vi "NT4 Format Generic  to String.vi"(9 "Quote Elements":bool, 11 "Variant":variant) -> (2 "Type String":string, 3 "String":string)   [LabVIEW 2025]
doc: "Format the generic union data into a string."
uses:
  <vilib>/Rock Robotics/Network Tables/NT Datatype.ctl
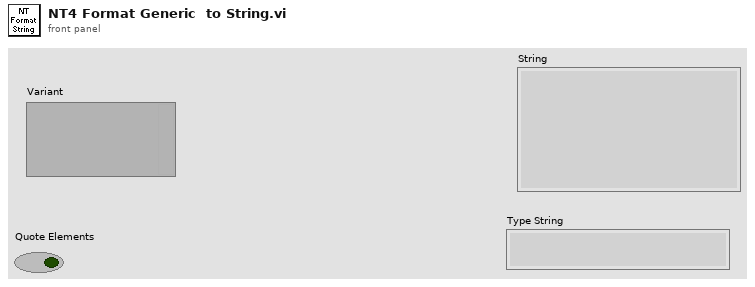
[diagram p1: front panel]
types:
  T1 = typedef "NT Datatype.ctl" = u32
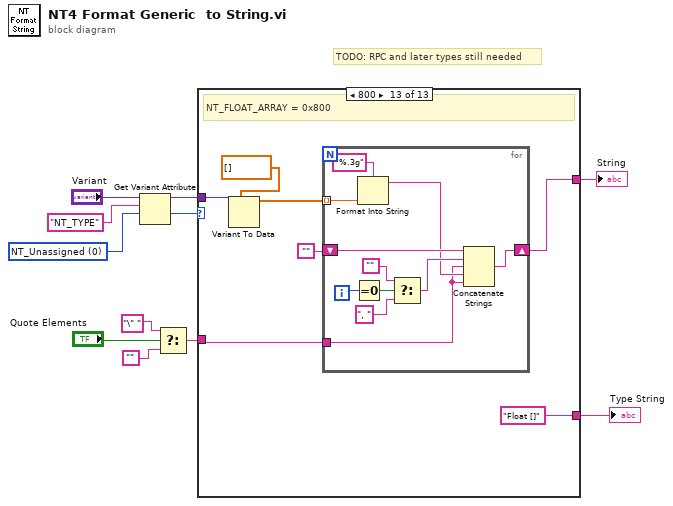
[diagram p0: block diagram]
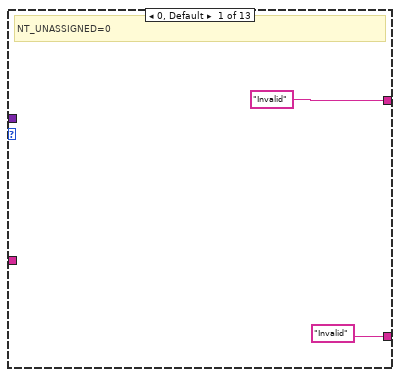
[diagram p2: hidden frame]
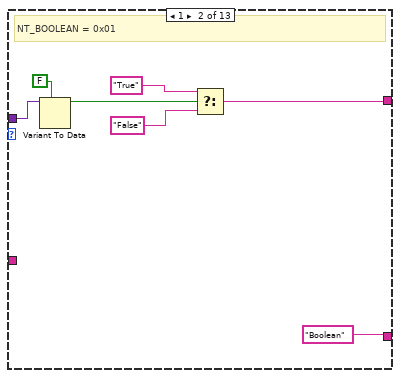
[diagram p3: hidden frame]
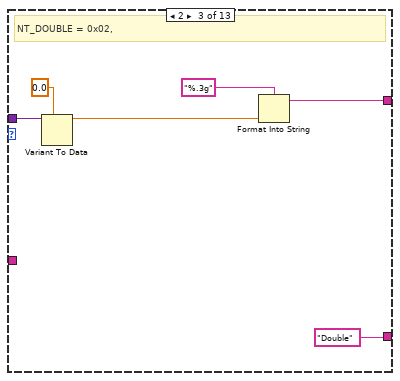
[diagram p4: hidden frame]
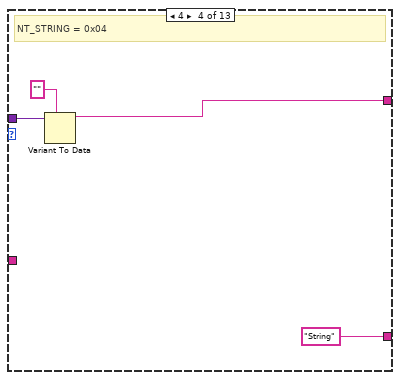
[diagram p5: hidden frame]
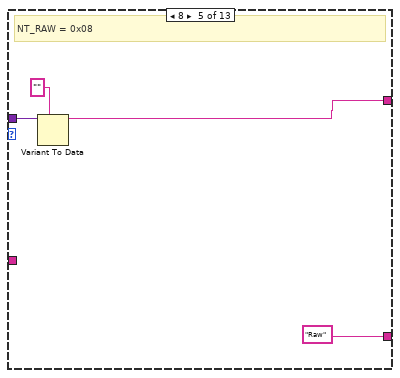
[diagram p6: hidden frame]
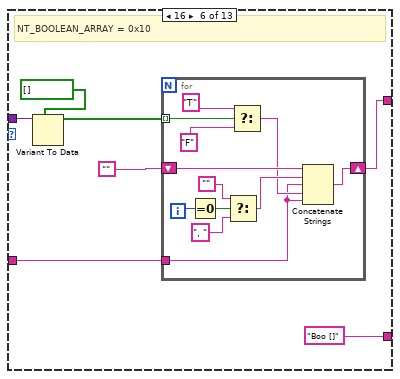
[diagram p7: hidden frame]
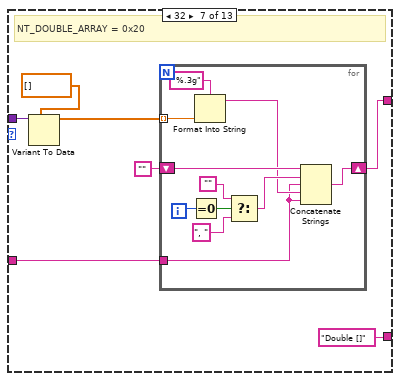
[diagram p8: hidden frame]
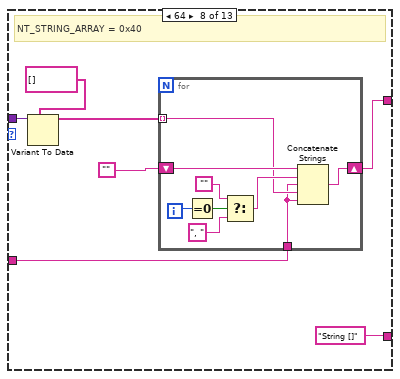
[diagram p9: hidden frame]
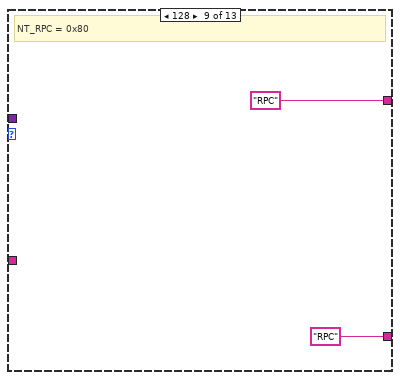
[diagram p10: hidden frame]
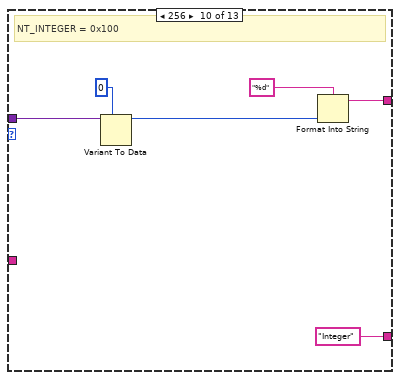
[diagram p11: hidden frame]
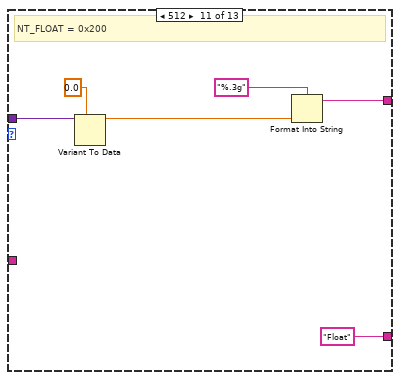
[diagram p12: hidden frame]
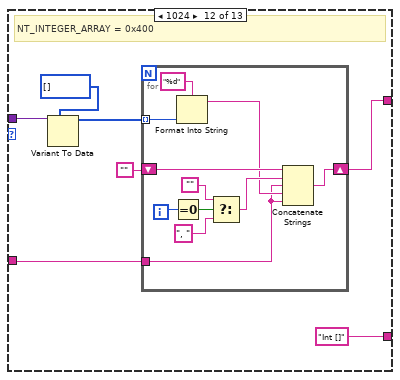
[diagram p13: hidden frame]
diagram:
  w2 = T1 0 items=["NT_Unassigned"=0, "NT_Boolean"=1, "NT_Double"=2, "NT_String"=4, "NT_Raw"=8, "NT_BooleanArray"=16, "NT_DoubleArray"=32, "NT_StringArray"=64, "NT_RPC"=128, "NT_Integer"=256, "NT_Float"=512, "NT_IntegerArray"=1024, "NT_FloatArray"=2048] ("NT_Type")
  # "TODO: RPC and later types still needed"
  n1 = Get Variant Attribute(Variant="Variant", name="NT_TYPE", default value (empty Variant)=w2) -> (duplicate Variant=w5:variant, value=w3:T1)  [unwired: 1 in, 2 out]
  n2 = Select(t="\" ", s="Quote Elements", f="") -> (s? t:f=w7:string)
  n3 = case shown="800" w3 {
    tunnel: ["Invalid" w18 w26 w29 w32 w40 w59 w77 "RPC" ("format string") w91 w97 w103 w121] -> w11
    tunnel: w7 -> [_ _ _ _ _ w39 w58 w76 _ _ _ w105 w122]
    tunnel: w5 -> [_ w17 w24 w30 w34 w38 w57 w75 _ w92 w98 w104 w123]
    tunnel: ["Invalid" "Boolean" "Double" "String" "Raw" "Boo []" "Double []" "String []" "RPC" "Integer" "Float" "Int []" "Float []"] -> w1
    frame 0, Default {
      # "NT_UNASSIGNED=0"
    }
    frame 1 {
      # "NT_BOOLEAN = 0x01"
      n4 = Variant To Data(type=FALSE ("Boolean"), Variant=w17) -> (data=w16:bool)  [unwired: 1 in, 1 out]
      n5 = Select(t="True", s=w16, f="False") -> (s? t:f=w18:string)
    }
    frame 2 {
      # "NT_DOUBLE = 0x02,"
      n6 = Variant To Data(type=0.0 ("input 1"), Variant=w24) -> (data=w23:dbl)  [unwired: 1 in, 1 out]
      n7 = Format Into String(format string="%.3g", w23) -> (resulting string=w26:string)  [unwired: 2 in, 1 out]
    }
    frame 4 {
      # "NT_STRING = 0x04"
      n8 = Variant To Data(type="" ("String"), Variant=w30) -> (data=w29:string)  [unwired: 1 in, 1 out]
    }
    frame 8 {
      # "NT_RAW = 0x08"
      n9 = Variant To Data(type="" ("String"), Variant=w34) -> (data=w32:string)  [unwired: 1 in, 1 out]
    }
    frame 16 {
      # "NT_BOOLEAN_ARRAY = 0x10"
      n10 = Variant To Data(type=bool[] [], Variant=w38) -> (data=w36:bool[])  [unwired: 1 in, 1 out]
      n11 = for {
        tunnel: w36 -> [w51] mode=indexing
        shift-right: [w44] -> w40
        shift-left: "" -> [w50]
        tunnel: w39 -> [w42]
        i -> [w49]
        n12 = Equal To 0?(x=w49) -> (x = 0?=w48:bool)
        n13 = Select(t="", s=w48, f=", ") -> (s? t:f=w45:string)
        n14 = Select(t="T", s=w51, f="F") -> (s? t:f=w43:string)
        n15 = Concatenate Strings(w50, w45, w42, w43, w42) -> (w44:string)
      }
    }
    frame 32 {
      # "NT_DOUBLE_ARRAY = 0x20"
      n16 = Variant To Data(type=dbl[] [], Variant=w57) -> (data=w55:dbl[])  [unwired: 1 in, 1 out]
      n17 = for {
        tunnel: w55 -> [w64] mode=indexing
        shift-right: [w65] -> w59
        shift-left: "" -> [w71]
        tunnel: w58 -> [w61]
        i -> [w70]
        n18 = Equal To 0?(x=w70) -> (x = 0?=w69:bool)
        n19 = Format Into String(format string="%.3g", w64) -> (resulting string=w62:string)  [unwired: 2 in, 1 out]
        n20 = Select(t="", s=w69, f=", ") -> (s? t:f=w66:string)
        n21 = Concatenate Strings(w71, w66, w61, w62, w61) -> (w65:string)
      }
    }
    frame 64 {
      # "NT_STRING_ARRAY = 0x40"
      n22 = Variant To Data(type=string[] [], Variant=w75) -> (data=w73:string[])  [unwired: 1 in, 1 out]
      n23 = for {
        tunnel: w73 -> [w80] mode=indexing
        shift-right: [w81] -> w77
        shift-left: "" -> [w87]
        tunnel: w76 -> [w79]
        i -> [w86]
        n24 = Equal To 0?(x=w86) -> (x = 0?=w85:bool)
        n25 = Select(t="", s=w85, f=", ") -> (s? t:f=w82:string)
        n26 = Concatenate Strings(w87, w82, w79, w80, w79) -> (w81:string)
      }
    }
    frame 128 {
      # "NT_RPC = 0x80"
    }
    frame 256 {
      # "NT_INTEGER = 0x100"
      n27 = Variant To Data(type=i64 0 ("input 1"), Variant=w92) -> (data=w95:i64)  [unwired: 1 in, 1 out]
      n28 = Format Into String(format string="%d", w95) -> (resulting string=w91:string)  [unwired: 2 in, 1 out]
    }
    frame 512 {
      # "NT_FLOAT = 0x200"
      n29 = Variant To Data(type=sgl 0.0 ("input 1"), Variant=w98) -> (data=w100:sgl)  [unwired: 1 in, 1 out]
      n30 = Format Into String(format string="%.3g", w100) -> (resulting string=w97:string)  [unwired: 2 in, 1 out]
    }
    frame 1024 {
      # "NT_INTEGER_ARRAY = 0x400"
      n31 = Variant To Data(type=i64[] [], Variant=w104) -> (data=w108:i64[])  [unwired: 1 in, 1 out]
      n32 = for {
        tunnel: w108 -> [w112] mode=indexing
        shift-right: [w113] -> w103
        shift-left: "" -> [w119]
        tunnel: w105 -> [w109]
        i -> [w118]
        n33 = Equal To 0?(x=w118) -> (x = 0?=w117:bool)
        n34 = Format Into String(format string="%d", w112) -> (resulting string=w110:string)  [unwired: 2 in, 1 out]
        n35 = Select(t="", s=w117, f=", ") -> (s? t:f=w114:string)
        n36 = Concatenate Strings(w119, w114, w109, w110, w109) -> (w113:string)
      }
    }
    frame 2048 {
      # "NT_FLOAT_ARRAY = 0x800"
      n37 = Variant To Data(type=sgl[] [], Variant=w123) -> (data=w126:sgl[])  [unwired: 1 in, 1 out]
      n38 = for {
        tunnel: w126 -> [w130] mode=indexing
        shift-right: [w131] -> w121
        shift-left: "" -> [w137]
        tunnel: w122 -> [w127]
        i -> [w136]
        n39 = Equal To 0?(x=w136) -> (x = 0?=w135:bool)
        n40 = Format Into String(format string="%.3g", w130) -> (resulting string=w128:string)  [unwired: 2 in, 1 out]
        n41 = Select(t="", s=w135, f=", ") -> (s? t:f=w132:string)
        n42 = Concatenate Strings(w137, w132, w127, w128, w127) -> (w131:string)
      }
    }
  }
  "String" <- w11
  "Type String" <- w1
